vi "Peek Message.vi"(8 "error in (no error)":errorcluster, 10 "Queue":string, 11 "Azure Session in":refnum<class "Session.lvclass">) -> (0 "error out":errorcluster, 2 "Message":T1, 3 "Azure Session out":refnum<class "Session.lvclass">)   [LabVIEW 2015, in "NI_Azure_Queue.lvlib"]
doc: "Retrieves a message from the front of the queue, without changing the message visibility."
uses:
  NI_Azure_Queue.lvlib
  Core/Session/Session.lvclass
  Message.ctl
  Core/Name Value Pair.ctl
  Core/Session/Session.lvclass/Session.ctl
  Core/Session/Write Request Parameters.vi
  Core/Session/Write HTTP Verb.vi
  Core/Session/Write URL Suffix.vi
  Core/NI_Azure_Core.lvlib
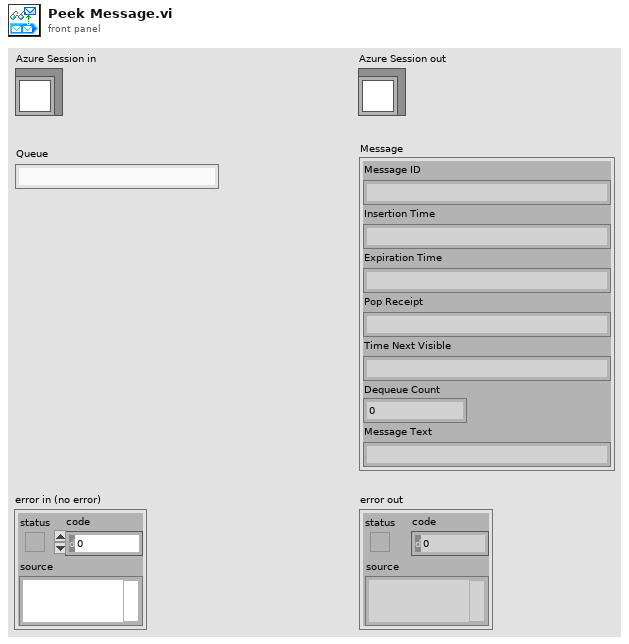
[diagram p1: front panel]
types:
  T1 = typedef "NI_Azure_Queue.lvlib/Message.ctl" = cluster{"Message ID":string, "Insertion Time":string, "Expiration Time":string, "Pop Receipt":string, "Time Next Visible":string, "Dequeue Count":i32, "Message Text":string}
  T2 = typedef "NI_Azure_Core.lvlib/Name Value Pair.ctl" = cluster{"name":string, "value":string}
  T3 = typedef "NI_Azure_Core.lvlib/Response.ctl" = cluster{"Headers":string, "Body":string}
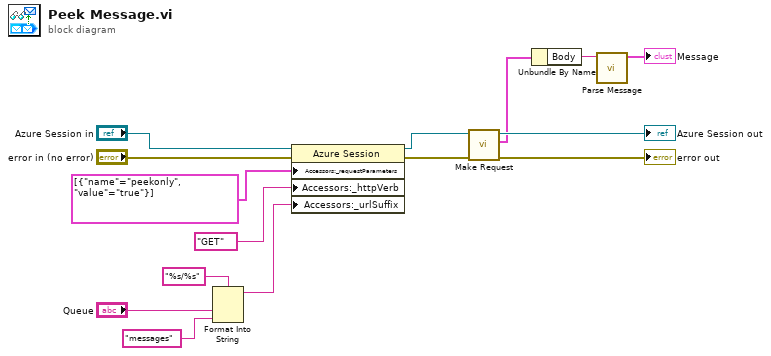
[diagram p0: block diagram]
diagram:
  n1 = Format Into String(format string="%s/%s", "Queue", "messages") -> (resulting string=w3:string)  [unwired: 2 in, 1 out]
  n2 = property class="Azure Session"(reference="Azure Session in", error in="error in (no error)", "Accessors:_requestParameters"=T2[] [{"name"="peekonly", "value"="true"}] ("request parameters"), "Accessors:_httpVerb"="GET" ("HTTP-Verb"), "Accessors:_urlSuffix"=w3) -> (reference out=w9:refnum<class "Session.lvclass">, error out=w11:errorcluster)
  n3 = call "Make Request.vi"("error in (no error)"=w11, "Session in"=w9) -> ("error out"=→"error out":errorcluster, "Response"=w12:T3, "Session out"=→"Azure Session out":refnum<class "Session.lvclass">)  [unwired: 7 in]
  n4 = Unbundle By Name(w12) -> ("Body"=w2:string)
  n5 = call "Parse Message.vi"("Body"=w2) -> ("Message"=→"Message":T1)  [unwired: 8 in, 2 out]
